vi "SR400 ReadStatus.vi"(6 "error in":errorcluster, 9 "Address string":string) -> (0 "Error Out":errorcluster, 3 "Status Code":u8)   [LabVIEW 2010]
uses:
  <vilib>/Utility/error.llb/DialogType.ctl
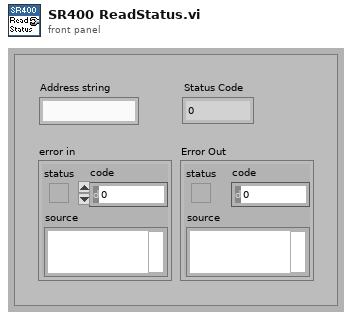
[diagram p1: front panel]
types:
  T1 = enum16{"Demande Statut", "Lit le Statut", "Oper. comp."}
  T2 = typedef "DialogType.ctl" = u16
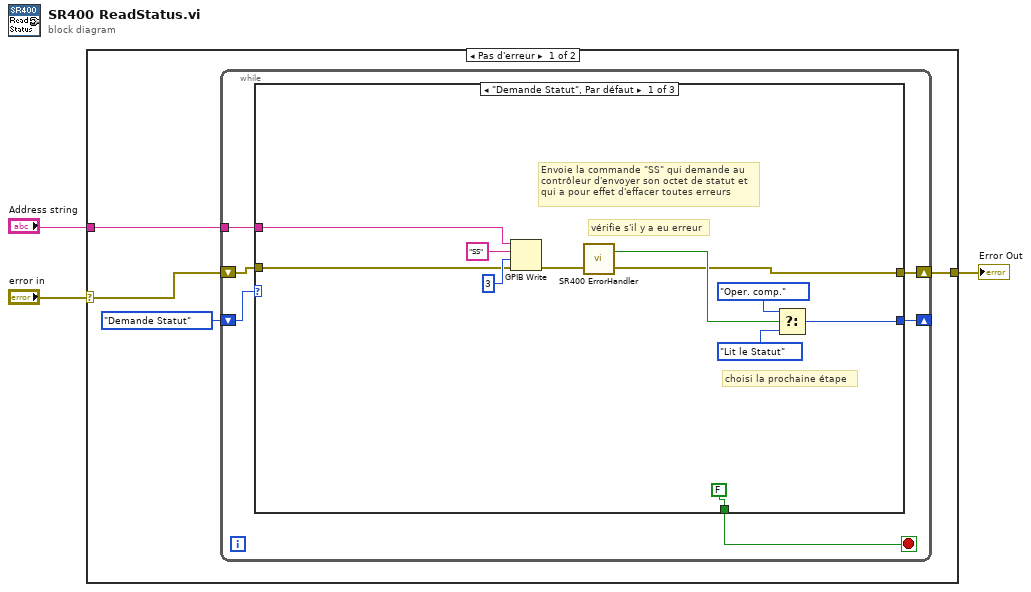
[diagram p0: block diagram]
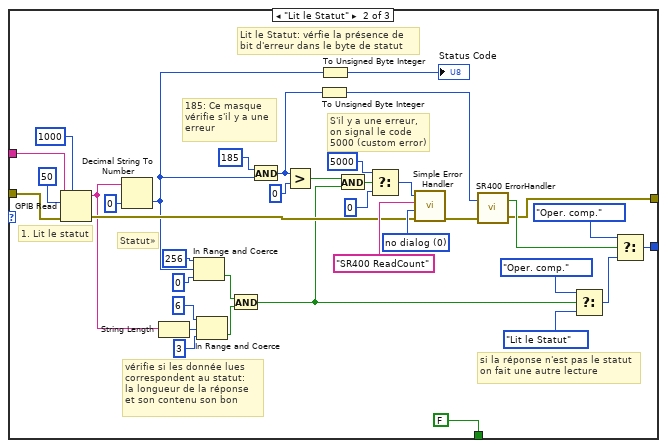
[diagram p2: hidden frame]
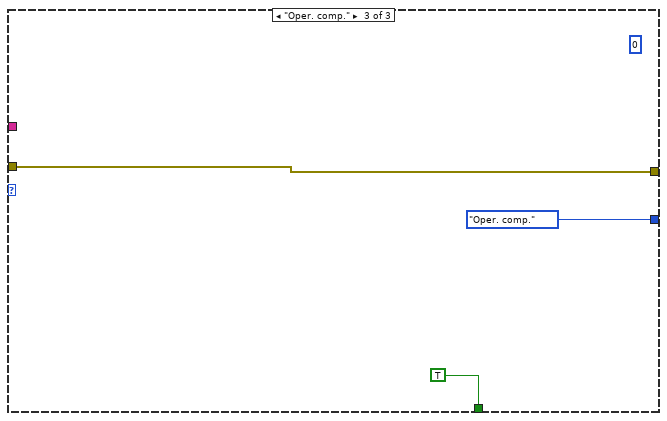
[diagram p3: hidden frame]
diagram:
  n1 = case shown="Pas d'erreur" "error in" {
    selector: "error in" -> [w6 w65]
    tunnel: "Address string" -> [w5 _]
    tunnel: [w4 w65] -> w1
    frame No Error {
      n2 = while {
        shift-right: [w13] -> _
        shift-left: T1."Demande Statut" -> [w12]
        shift-right: [w9] -> w4
        shift-left: w6 -> [w11]
        tunnel: w5 -> [w10]
        stop <- w8 stop-if-true
        n3 = case shown="\"Demande Statut\", Par défaut" w12 {
          tunnel: [w18 w32 T1."Oper. comp."] -> w13
          tunnel: w11 -> [w17 w35 w62]
          tunnel: w10 -> [w16 w34 _]
          tunnel: [w15 w28 w62] -> w9
          tunnel: [FALSE FALSE ("Données lues") TRUE] -> w8
          frame "Demande Statut", Default {
            # "choisi la prochaine étape"
            # "vérifie s'il y a eu erreur"
            # "Envoie la commande \"SS\" qui demande au contrôleur d'envoyer son octet de statut et qui a pour effet d'effacer toutes erreurs"
            n4 = GPIB Write(0:w16, 1:"SS" ("data"), 2:i16 3 ("mode (0)"), 3:w17) -> (6:w22:errorcluster)  [unwired: 1 in, 1 out]
            n5 = call <userlib>:"SR400 ErrorHandler.vi"("error in (no error)"=w22) -> ("error out"=w15:errorcluster, "Erreur"=w21:bool)  [unwired: 1 in]
            n6 = Select(t=T1."Oper. comp.", s=w21, f=T1."Lit le Statut") -> (s? t:f=w18:T1)
          }
          frame "Lit le Statut" {
            w57 = T2 0 items=["no dialog", "OK message", "continue or stop message", "OK message + warnings", "continue/stop + warnings"] ("type of dialog (OK msg:1)")
            # "Statut»"
            # "1. Lit le statut"
            # "si la réponse n'est pas le statut\non fait une autre lecture"
            # "vérifie si les donnée lues correspondent au statut:\nla longueur de la réponse  et son contenu son bon"
            # "S'il y a une erreur, on signal le code 5000 (custom error)"
            # "Lit le Statut: vérfie la présence de bit d'erreur dans le byte de statut"
            # "185: Ce masque vérifie s'il y a une erreur"
            n7 = GPIB Read(0:w34, 1:50 ("byte count"), 3:w35, 4:1000 ("timeout ms (488.2 global)")) -> (5:w48:string, 7:w51:errorcluster)  [unwired: 1 in, 1 out]
            n8 = Decimal String To Number(string=w48, default (0L)=i16 0 ("default (0 I32)")) -> (number=w25:i16)  [unwired: 1 in, 1 out]
            n9 = String Length(string=w48) -> (length=w40:i32)
            n10 = In Range and Coerce(upper limit=i16 256, x=w25, lower limit=i16 0) -> (In Range?=w46:bool)  [unwired: 1 out]
            n11 = In Range and Coerce(upper limit=6 ("y"), x=w40, lower limit=3 ("y")) -> (In Range?=w37:bool)  [unwired: 1 out]
            n12 = And(x=w46, y=w37) -> (x .and. y?=w43:bool)
            n13 = And(x=i16 185, y=w25) -> (x .and. y?=w54:i16)
            n14 = Greater?(x=w54, y=i16 0) -> (0:w45:bool)
            n15 = To Unsigned Byte Integer(number=w54) -> (unsigned 8bit integer=w53:u8)
            n16 = To Unsigned Byte Integer(number=w25) -> (unsigned 8bit integer=→"Status Code":u8)
            n17 = And(x=w45, y=w43) -> (x .and. y?=w44:bool)
            n18 = Select(t=5000, s=w44, f=0) -> (s? t:f=w58:i32)
            n19 = call <vilib>:"Simple Error Handler.vi"("error code (no error:0)"=w58, "error source (\" \")"="SR400 ReadCount" ("[error source] (\" \")"), "type of dialog (OK msg:1)"=w57, "error in (no error)"=w51) -> ("error out"=w55:errorcluster)  [unwired: 1 in, 4 out]
            n20 = call <userlib>:"SR400 ErrorHandler.vi"("error in (no error)"=w55, "Status Code"=w53) -> ("error out"=w28:errorcluster, "Erreur"=w42:bool)
            n21 = Select(t=T1."Oper. comp.", s=w43, f=T1."Lit le Statut") -> (s? t:f=w41:T1)
            n22 = Select(t=T1."Oper. comp.", s=w42, f=w41) -> (s? t:f=w32:T1)
          }
          frame "Oper. comp." {
            (unwired) u8 0
          }
        }
      }
    }
    frame Error {
    }
  }
  "Error Out" <- w1
